vi "http get all headers and fields.vi"(11 "headers":T1) -> (2 "data":string[](array[string]), 3 "fields":string[](array[string]))   [LabVIEW 2013, in "http headers.lvlib"]
uses:
  http headers.lvlib
  http header data.ctl
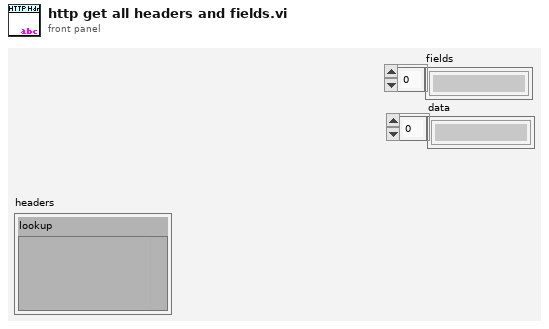
[diagram p1: front panel]
types:
  T1 = typedef "http headers.lvlib/http header data.ctl" = cluster{"lookup":variant}
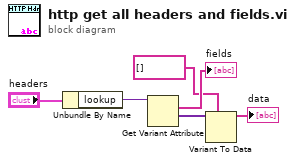
[diagram p0: block diagram]
diagram:
  n1 = Unbundle By Name("headers") -> ("lookup"=w5:variant)
  n2 = Get Variant Attribute(Variant=w5) -> (names=→"fields":string[], values=w3:variant[])  [unwired: 3 in, 2 out]
  n3 = Variant To Data(type=string[] [] ("names"), Variant=w3) -> (data=→"data":string[])  [unwired: 1 in, 1 out]
